vi "S2C_ExeLoopStatus.vi"(8 "Error In":errorcluster, 11 "Reset?":bool) -> (0 "Error Out":errorcluster)   [LabVIEW 2015]
doc: "Sets the cell background and font color for the execution table results cell."
uses:
  Globals/S2C_Globals.vi
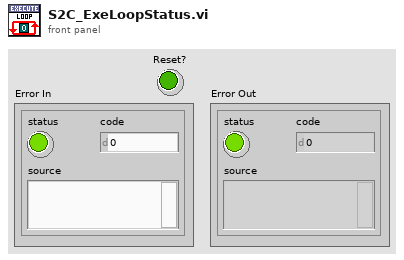
[diagram p1: front panel]
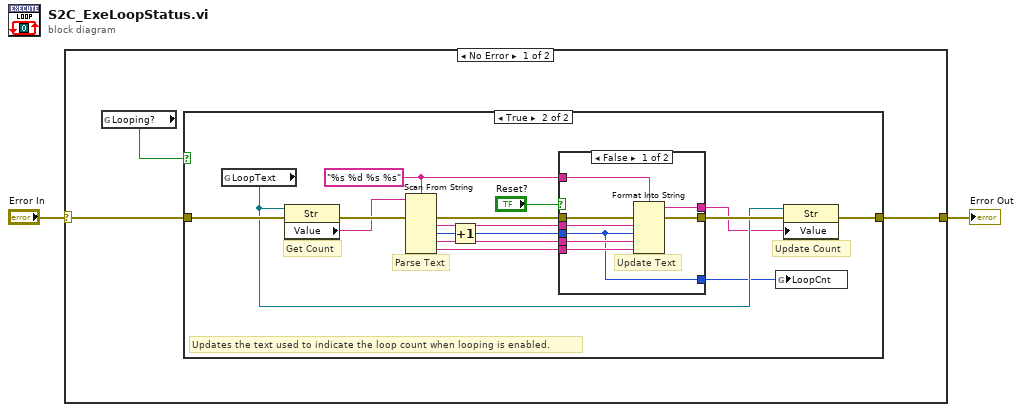
[diagram p0: block diagram]
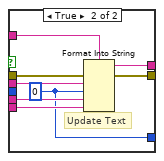
[diagram p3: hidden frame]
diagram:
  n1 = case shown="No Error" "Error In" {
    selector: "Error In" -> [w5 w39]
    tunnel: [w3 w39] -> w1
    frame No Error {
      n2 = global read "S2C_Globals.vi" "Looping?"() -> (w4:bool)
      n3 = case shown="True" w4 {
        tunnel: w5 -> [w6 w22]
        tunnel: [w6 w10] -> w3
        frame False {
          # "Looping not enabled"
        }
        frame True {
          w16 = "%s %d %s %s" ("format string")
          # "Updates the text used to indicate the loop count when looping is enabled."
          # "Parse Text"
          # "Update Count"
          # "Get Count"
          n4 = global read "S2C_Globals.vi" "LoopText"() -> (w12:refnum<vi>)
          n5 = property class="Str"(reference=w12, error in=w22) -> (error out=w15:errorcluster, "Value"=w14:string)  [unwired: 1 out]
          n6 = Scan From String(format string=w16, input string=w14, error in=w15) -> (error out=w17:errorcluster, output 1=w20:string, output 2=w21:i32, output 3=w19:string, output 4=w18:string)  [unwired: 5 in, 2 out]
          n7 = Increment(x=w21) -> (x+1=w8:i32)
          n8 = case shown="False" "Reset?" {
            tunnel: w20 -> [w30 w38]
            tunnel: w8 -> [w23 _]
            tunnel: w19 -> [w29 w37]
            tunnel: w18 -> [w28 w36]
            tunnel: w17 -> [w27 w35]
            tunnel: w16 -> [w26 w34]
            tunnel: [w25 w33] -> w13
            tunnel: [w24 w32] -> w11
            tunnel: [w23 w31] -> w7
            frame False {
              # "Update Text"
              n9 = Format Into String(format string=w26, error in=w27, w30, w23, w29, w28) -> (resulting string=w24:string, error out=w25:errorcluster)  [unwired: 1 in]
            }
            frame True {
              w31 = 0 ("input 2")
              # "Update Text"
              n10 = Format Into String(format string=w34, error in=w35, w38, w31, w37, w36) -> (resulting string=w32:string, error out=w33:errorcluster)  [unwired: 1 in]
            }
          }
          n11 = global write "S2C_Globals.vi" "LoopCnt"(w7) -> ()
          n12 = property class="Str"(reference=w12, error in=w13, "Value"=w11) -> (error out=w10:errorcluster)  [unwired: 1 out]
        }
      }
    }
    frame Error {
    }
  }
  "Error Out" <- w1
